vi "aft_LMS_Check_Configurations.vi"(8 "error in (no error)":errorcluster, 11 "fixed-point LMS settings":T1) -> (0 "error out":errorcluster)   [LabVIEW 2017, in "NI_AdaptiveFilter.lvlib"]
uses:
  <vilib>/addons/Adaptive Filters/NI_AdaptiveFilter.lvlib
  <vilib>/addons/Adaptive Filters/Utilities/AFT Errors.ctl
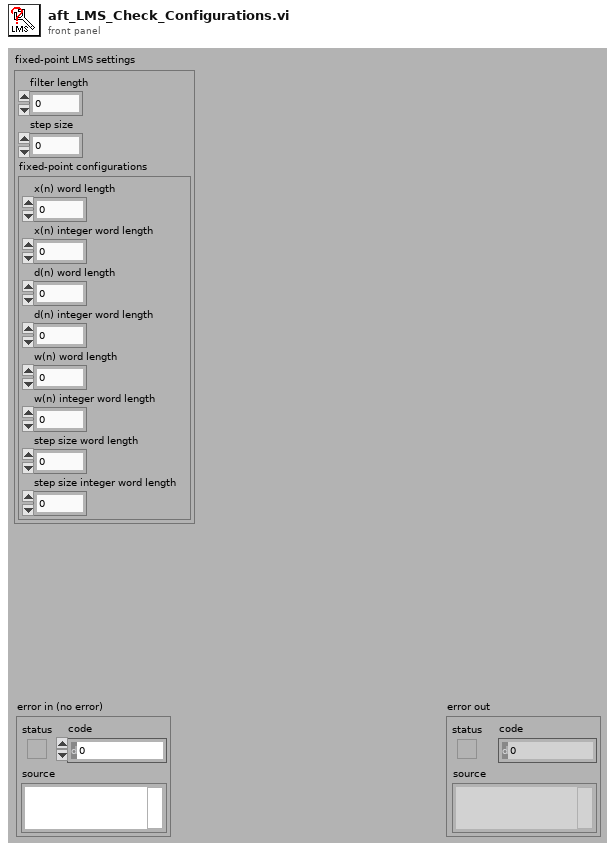
[diagram p1: front panel]
types:
  T1 = cluster{"filter length":i32, "step size":dbl, "fixed-point configurations":cluster{"x(n) word length":i32, "x(n) integer word length":i32, "d(n) word length":i32, "d(n) integer word length":i32, "w(n) word length":i32, "w(n) integer word length":i32, "step size word length":i32, "step size integer word length":i32}}
  T2 = typedef "NI_AdaptiveFilter.lvlib/AFT Errors.ctl" = i32
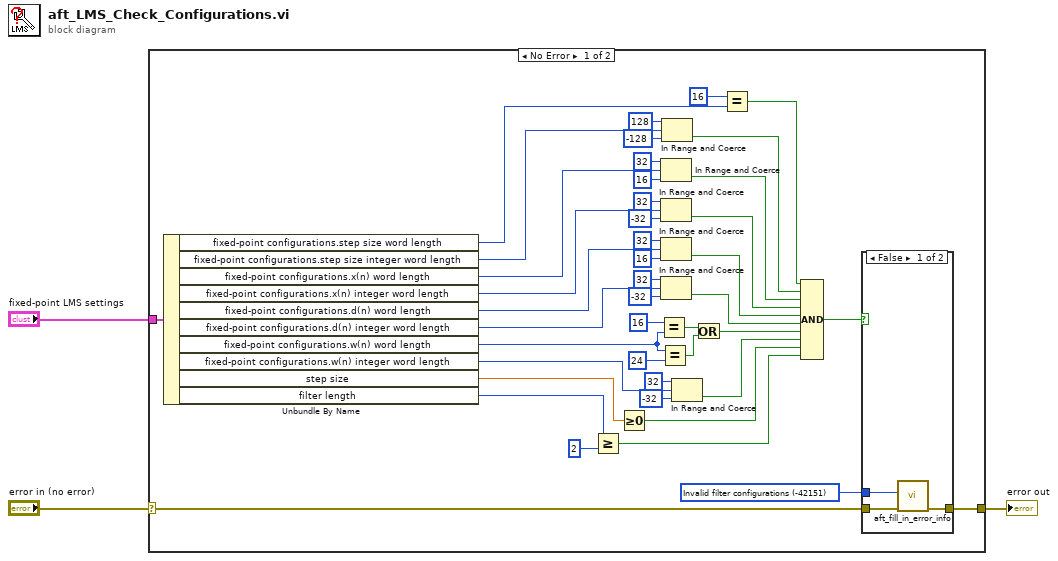
[diagram p0: block diagram]
diagram:
  n1 = case shown="No Error" "error in (no error)" {
    selector: "error in (no error)" -> [w42 w51]
    tunnel: "fixed-point LMS settings" -> [w46 _]
    tunnel: [w41 w51] -> w2
    frame No Error {
      w4 = T2 -42151 items=["No errors"=0, "No valid FPGA target"=-42150, "Invalid filter configurations"=-42151, "LabVIEW FPGA or NI-RIO not installed"=-42152, "File exists on disk"=-42153, "File exists in memory"=-42154] ("AFT errors")
      n2 = Unbundle By Name(w46) -> ("fixed-point configurations.step size word length"=w11:i32, "fixed-point configurations.step size integer word length"=w9:i32, "fixed-point configurations.x(n) word length"=w40:i32, "fixed-point configurations.x(n) integer word length"=w37:i32, "fixed-point configurations.d(n) word length"=w30:i32, "fixed-point configurations.d(n) integer word length"=w29:i32, "fixed-point configurations.w(n) word length"=w23:i32, "fixed-point configurations.w(n) integer word length"=w26:i32, "step size"=w45:dbl, "filter length"=w43:i32)
      n3 = Greater Or Equal?(x=w43, y=2) -> (x >= y?=w13:bool)
      n4 = Greater Or Equal To 0?(x=w45) -> (x >= 0?=w14:bool)
      n5 = Equal?(x=16 ("y"), y=w23) -> (x = y?=w22:bool)
      n6 = Equal?(x=w23, y=24) -> (x = y?=w21:bool)
      n7 = In Range and Coerce(upper limit=32, x=w40, lower limit=16) -> (In Range?=w20:bool)  [unwired: 1 out]
      n8 = In Range and Coerce(upper limit=32, x=w37, lower limit=-32) -> (In Range?=w19:bool)  [unwired: 1 out]
      n9 = In Range and Coerce(upper limit=32, x=w30, lower limit=16) -> (In Range?=w18:bool)  [unwired: 1 out]
      n10 = In Range and Coerce(upper limit=32, x=w29, lower limit=-32) -> (In Range?=w17:bool)  [unwired: 1 out]
      n11 = In Range and Coerce(upper limit=128, x=w9, lower limit=-128) -> (In Range?=w6:bool)  [unwired: 1 out]
      n12 = In Range and Coerce(upper limit=32, x=w26, lower limit=-32) -> (In Range?=w15:bool)  [unwired: 1 out]
      n13 = Or(x=w22, y=w21) -> (x .or. y?=w16:bool)
      n14 = Equal?(x=16, y=w11) -> (x = y?=w5:bool)
      n15 = Compound Arithmetic op=AND(w5, w6, w20, w19, w18, w17, w16, w15, w14, w13) -> (w12:bool)
      n16 = case shown="False" w12 {
        tunnel: w42 -> [w48 w50]
        tunnel: [w49 w50] -> w41
        tunnel: w4 -> [w47 _]
        frame False {
          n17 = call <vilib>:"aft_fill_in_error_info.vi"("error in"=w48, "status code"=w47) -> ("error out"=w49:errorcluster)  [unwired: 2 in, 7 out]
        }
        frame True {
        }
      }
    }
    frame Error {
    }
  }
  "error out" <- w2
